vi "SR1-Test.vi"() -> ()   [LabVIEW 2014]
uses:
  Stanford Research SR1.lvlib
panel:
  in  "Start Button":bool
  out "Spectrum":cluster{dbl, dbl, dbl[]}(graph)
  in  "Read Button":bool
  in  "Stop Button":bool
  out "error out":errorcluster
  out "ID":string
  in  "VISA resource name":refnum<visa-resource-name>
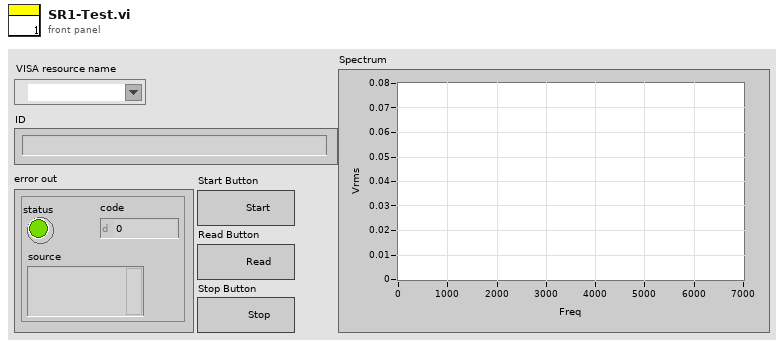
[diagram p1: front panel]
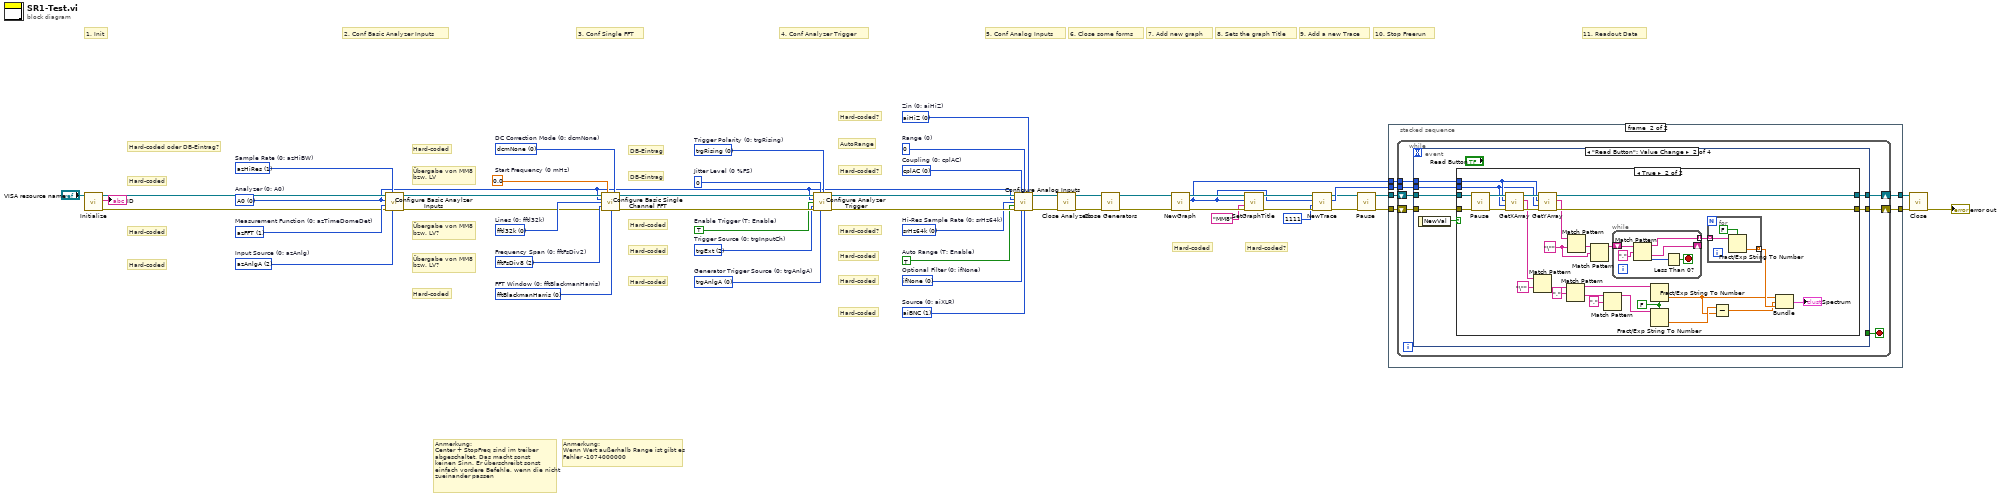
[diagram p0: block diagram]
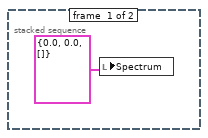
[diagram p2: hidden frame]
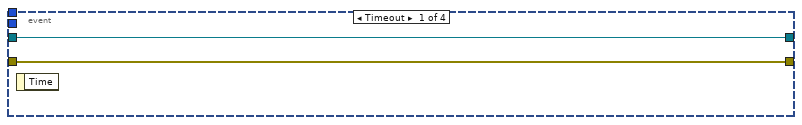
[diagram p3: hidden frame]
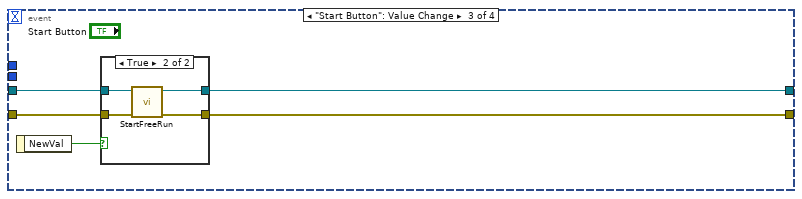
[diagram p5: hidden frame]
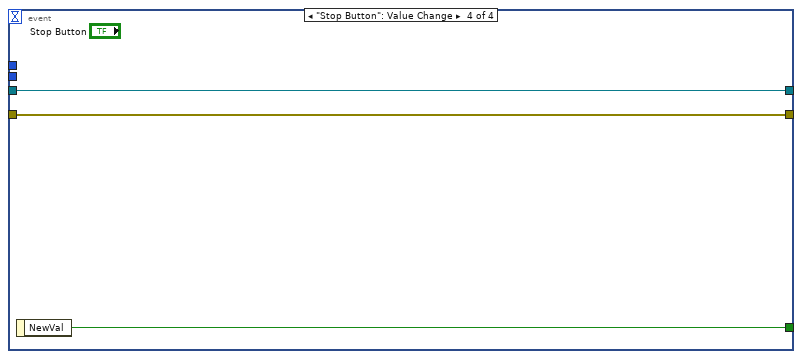
[diagram p7: hidden frame]
diagram:
  w22 = 0 items=["aiHiZ", "aiz300", "aiz600"]  # Zin (0: aiHiZ)
  w23 = 0  # Range (0)
  w24 = u16 0 items=["cplAC", "cplDC"]  # Coupling (0: cplAC)
  w25 = 1 items=["aiXLR", "aiBNC", "aiGenMon", "aiDigCommonMode"]  # Source (0: aiXLR)
  w26 = 0 items=["ifNone", "ifFiler1", "ifFilter2", "ifFilter3", "ifFilter4", "ifGround"]  # Optional Filter (0: ifNone)
  w27 = 0 items=["srHz64k", "srHz128k", "srOSR", "srOSRx2"]  # Hi-Res Sample Rate (0: srHz64k)
  w28 = TRUE  # Auto Range (T: Enable)
  w31 = 0 items=["trgAnlgA", "trgAnlgB", "trgDigA", "trgDigB", "trgJitter"]  # Generator Trigger Source (0: trgAnlgA)
  w32 = 2 items=["trgInputCh", "trgOtherCh", "trgExt", "trgManual", "trgGen", "trgDigAudBlock", "trgBurstA", "trgBurstB"]  # Trigger Source (0: trgInputCh)
  w33 = u16 0 items=["trgRising", "trgFalling"]  # Trigger Polarity (0: trgRising)
  w34 = 0  # Jitter Level (0 %FS)
  w35 = TRUE  # Enable Trigger (T: Enable)
  w40 = 1 items=["azHiBW", "azHiRes", "azISR", "azDetOutSR"]  # Sample Rate (0: azHiBW)
  w41 = 2 items=["azAnlg", "azDig", "azAnlgA", "azAnlgB", "azDigA", "azDigB", "azDetOut"]  # Input Source (0: azAnlg)
  w21 = 0 items=["A0", "A1"]  # Analyzer (0: A0)
  w42 = 1 items=["azTimeDomeDet", "azFFT", "azFFT2Ch", "azTHD", "azIMD", "azMultitone", "azJitter", "azHistogram", "azOctave"]  # Measurement Function (0: azTimeDomeDet)
  w45 = 0 items=["dcmNone", "dcmMean", "dcmPkPK"]  # DC Correction Mode (0: dcmNone)
  w46 = 0 items=["fftBlackmanHarris", "fftHann", "fftHamming", "fftEquiripple", "fftFlattop", "fftGaussian", "fftKaiser", "fftUniform", "fftRifeVincent4", "fftRifeVincent5", "fftRifeVincent10", "fftBlackmanHarris7", "fftVariable"]  # FFT Window (0: fftBlackmanHarris)
  w47 = 2 items=["fftFsDiv2", "fftFsDiv4", "fftFsDiv8", "fftFsDiv16", "fftFsDiv32", "fftFsDiv64", "fftFsDiv128", "fftFsDiv256", "fftFsDiv512", "fftFsDiv1024"]  # Frequency Span (0: fftFsDiv2)
  w48 = 0 items=["fftl32k", "fftl16k", "fftl8k", "fftl4k", "fftl2k", "fftl1k", "fftl512", "fftl256"]  # Lines (0: fftl32k)
  w49 = 0.0  # Start Frequency (0 mHz)
  # "11. Readout Data"
  # "10. Stop Freerun"
  # "Hard-coded"
  # "Hard-coded?"
  # "9. Add a new Trace"
  # "8. Sets the graph Title"
  # "7. Add new graph"
  # "6. Close some forms"
  # "5. Conf Analog Inputs"
  # "4. Conf Analyzer Trigger"
  # "3. Conf Single FFT"
  # "2. Conf Basic Analyzer Inputs"
  # "1. Init"
  # "Hard-coded"
  # "Hard-coded"
  # "Hard-coded"
  # "Hard-coded?"
  # "Hard-coded?"
  # "AutoRange"
  # "Hard-coded?"
  # "Hard-coded"
  # "Hard-coded"
  # "Hard-coded"
  # "DB-Eintrag"
  # "DB-Eintrag"
  # "Hard-coded"
  # "Übergabe von MM8\nbzw. LV?"
  # "Übergabe von MM8\nbzw. LV?"
  # "Übergabe von MM8\nbzw. LV"
  # "Hard-coded"
  # "Hard-coded"
  # "Hard-coded"
  # "Hard-coded"
  # "Hard-coded oder DB-Eintrag?"
  # "Anmerkung:\nWenn Wert außerhalb Range ist gibt es\nFehler -1074000000"
  # "Anmerkung:\nCenter + StopFreq sind im treiber\nabgeschaltet. Das macht sonst \nkeinen Sinn. Er überschreibt sonst\neinfach vordere Befehle, wenn die nicht\nzueinander passen"
  n1 = call "Initialize.vi"("VISA resource name"="VISA resource name") -> ("error out"=w38:errorcluster, "ID"=→"ID":string, "VISA resource name out"=w39:refnum<visa-resource-name>)  [unwired: 8 in]
  n2 = call "Configure Basic Anaylzer Inputs.vi"("Input Source (0: azAnlg)"=w41, "Sample Rate (0: azHiBW)"=w40, "error in (no error)"=w38, "Measurement Function (0: azTimeDomeDet)"=w42, "Analyzer (0: A0)"=w21, "VISA resource name"=w39) -> ("error out"=w44:errorcluster, "VISA resource name out"=w43:refnum<visa-resource-name>)  [unwired: 4 in]
  n3 = call "Configure Basic Single Channel FFT .vi"("VISA resource name"=w43, "Start Frequency (0 mHz)"=w49, "DC Correction Mode (0: dcmNone)"=w45, "Analyzer (0: A0)"=w21, "Lines (0: fftl32k)"=w48, "Frequency Span (0: fftFsDiv2)"=w47, "error in (no error)"=w44, "FFT Window (0: fftBlackmanHarris)"=w46) -> ("VISA resource name out"=w36:refnum<visa-resource-name>, "error out"=w37:errorcluster)  [unwired: 6 in]
  n4 = call "Configure Analyzer Trigger.vi"("VISA resource name"=w36, "Jitter Level (0 %FS)"=w34, "Trigger Polarity (0: trgRising)"=w33, "Analyzer (0: A0)"=w21, "Enable Trigger (T: Enable)"=w35, "Trigger Source (0: trgInputCh)"=w32, "error in (no error)"=w37, "Generator Trigger Source (0: trgAnlgA)"=w31) -> ("VISA resource name out"=w29:refnum<visa-resource-name>, "error out"=w30:errorcluster)  [unwired: 6 in]
  n5 = call "Configure Analog Inputs.vi"("VISA resource name"=w29, "Coupling (0: cplAC)"=w24, "Range (0)"=w23, "Zin (0: aiHiZ)"=w22, "Channel (0: ChannelA)"=w21, "Hi-Res Sample Rate (0: srHz64k)"=w27, "Auto Range (T: Enable)"=w28, "error in (no error)"=w30, "Optional Filter (0: ifNone)"=w26, "Source (0: aiXLR)"=w25) -> ("VISA resource name out"=w18:refnum<visa-resource-name>, "error out"=w17:errorcluster)  [unwired: 4 in]
  n6 = call "Close Analyzers.vi"("error in (no error)"=w17, "VISA resource name"=w18) -> ("error out"=w20:errorcluster, "VISA resource name out"=w19:refnum<visa-resource-name>)  [unwired: 8 in]
  n7 = call "Close Generators.vi"("error in (no error)"=w20, "VISA resource name"=w19) -> ("error out"=w16:errorcluster, "VISA resource name out"=w15:refnum<visa-resource-name>)  [unwired: 8 in]
  n8 = call "NewGraph.vi"("error in (no error)"=w16, "VISA resource name"=w15) -> ("error out"=w12:errorcluster, "GraphID"=w6:i32, "VISA resource name out"=w11:refnum<visa-resource-name>)  [unwired: 7 in]
  n9 = call "SetGraphTitle.vi"("error in (no error)"=w12, "Title"="MM8", "GraphID"=w6, "VISA resource name"=w11) -> ("error out"=w13:errorcluster, "VISA resource name out"=w14:refnum<visa-resource-name>)  [unwired: 6 in]
  n10 = call "NewTrace.vi"("error in (no error)"=w13, "TraceType"=1111, "GraphID"=w6, "VISA resource name"=w14) -> ("error out"=w4:errorcluster, "TraceID"=w5:i32, "VISA resource name out"=w2:refnum<visa-resource-name>)  [unwired: 5 in]
  n11 = call "Pause.vi"("error in (no error)"=w4, "VISA resource name"=w2) -> ("error out"=w3:errorcluster, "VISA resource name out"=w1:refnum<visa-resource-name>)  [unwired: 8 in]
  n12 = stacked-sequence {
    tunnel: [_ w59] -> w8
    tunnel: [_ w58] -> w7
    tunnel: w6 -> [_ w57]
    tunnel: w5 -> [_ w56]
    tunnel: w3 -> [_ w55]
    tunnel: w1 -> [_ w54]
    frame #0 {
      n13 = local write "Spectrum"(cluster{dbl, dbl, dbl[]} {0.0, 0.0, []} ("Spectrum")) -> ()
    }
    frame #1 {
      n14 = while {
        shift-right: [w63] -> w58
        shift-left: w54 -> [w62]
        shift-right: [w64] -> w59
        shift-left: w55 -> [w65]
        tunnel: w57 -> [w61]
        tunnel: w56 -> [w60]
        stop <- w66 stop-if-true
        n15 = event shown="[1] \"Read Button\": Value Change" {
          selector: _ -> [_ _ _ _]
          dyn-events: _ -> [_ _ _ _]
          timeout: _ -> [_ _ _ _]
          tunnel: [_ _ _ w129] -> w66
          tunnel: w65 -> [w68 w74 w119 w128]
          tunnel: [w68 w72 w116 w128] -> w64
          tunnel: [w67 w71 w117 w127] -> w63
          tunnel: w62 -> [w67 w73 w120 w127]
          tunnel: w61 -> [_ w70 _ _]
          tunnel: w60 -> [_ w69 _ _]
          event Timeout {
            n16 = event-data() -> ()  [unwired: 1 in, 1 out]
          }
          event "Read Button": Value Change {
            n17 = event-data() -> ("NewVal"=w75:bool)  [unwired: 1 in]
            n18 = case shown="True" w75 {
              tunnel: w74 -> [w76 w106]
              tunnel: w73 -> [w77 w105]
              tunnel: [w76 w101] -> w72
              tunnel: [w77 w99] -> w71
              tunnel: w70 -> [_ w98]
              tunnel: w69 -> [_ w97]
              frame False {
              }
              frame True {
                w83 = FALSE ("use system decimal point (T)")
                w96 = "\"" ("regular expression")
                n19 = call "Pause.vi"("error in (no error)"=w106, "VISA resource name"=w105) -> ("error out"=w103:errorcluster, "VISA resource name out"=w104:refnum<visa-resource-name>)  [unwired: 8 in]
                n20 = call "GetXArray.vi"("error in (no error)"=w103, "TraceID"=w97, "GraphID"=w98, "VISA resource name"=w104) -> ("error out"=w102:errorcluster, "xArray"=w90:string, "VISA resource name out"=w100:refnum<visa-resource-name>)  [unwired: 5 in]
                n21 = Match Pattern(string=w90, regular expression="\"") -> (after substring=w89:string)  [unwired: 1 in, 3 out]
                n22 = call "GetYArray.vi"("error in (no error)"=w102, "TraceID"=w97, "GraphID"=w98, "VISA resource name"=w100) -> ("error out"=w101:errorcluster, "yArray"=w93:string, "VISA resource name out"=w99:refnum<visa-resource-name>)  [unwired: 5 in]
                n23 = Match Pattern(string=w89, regular expression=",") -> (before substring=w85:string, after substring=w86:string)  [unwired: 1 in, 2 out]
                n24 = Match Pattern(string=w93, regular expression=w96) -> (after substring=w94:string)  [unwired: 1 in, 3 out]
                n25 = Match Pattern(string=w94, regular expression=w96) -> (before substring=w95:string)  [unwired: 1 in, 3 out]
                n26 = Match Pattern(string=w86, regular expression=",") -> (before substring=w84:string)  [unwired: 1 in, 3 out]
                n27 = while {
                  tunnel: [w110] -> w92 mode=indexing
                  shift-right: [w109] -> _
                  shift-left: w95 -> [w112]
                  stop <- w107 stop-if-true
                  n28 = Match Pattern(string=w112, regular expression=",") -> (before substring=w110:string, after substring=w109:string, offset past match=w108:i32)  [unwired: 1 in, 1 out]
                  n29 = Less Than 0?(x=w108) -> (x < 0?=w107:bool)
                }
                n30 = Fract/Exp String To Number(use system decimal point (T)=w83, string=w85) -> (number=w79:dbl)  [unwired: 2 in, 1 out]
                n31 = Fract/Exp String To Number(use system decimal point (T)=w83, string=w84) -> (number=w80:dbl)  [unwired: 2 in, 1 out]
                n32 = for {
                  tunnel: w92 -> [w115] mode=indexing
                  tunnel: [w113] -> w82 mode=indexing
                  n33 = Fract/Exp String To Number(use system decimal point (T)=FALSE, string=w115) -> (number=w113:dbl)  [unwired: 2 in, 1 out]
                }
                n34 = Subtract(x=w80, y=w79) -> (x-y=w78:dbl)
                n35 = Bundle(w79, w78, w82) -> (→"Spectrum":cluster{dbl, dbl, dbl[]})  [unwired: 1 in]
              }
            }
          }
          event "Start Button": Value Change {
            n36 = event-data() -> ("NewVal"=w118:bool)  [unwired: 1 in]
            n37 = case shown="True" w118 {
              tunnel: w120 -> [w122 w126]
              tunnel: w119 -> [w121 w125]
              tunnel: [w122 w124] -> w117
              tunnel: [w121 w123] -> w116
              frame False {
              }
              frame True {
                n38 = call "StartFreeRun.vi"("error in (no error)"=w125, "VISA resource name"=w126) -> ("error out"=w123:errorcluster, "VISA resource name out"=w124:refnum<visa-resource-name>)  [unwired: 8 in]
              }
            }
          }
          event "Stop Button": Value Change {
            n39 = event-data() -> ("NewVal"=w129:bool)  [unwired: 1 in]
          }
        }
      }
    }
  }
  n40 = call "Close.vi"("error in (no error)"=w8, "VISA resource name"=w7) -> ("error out"=→"error out":errorcluster)  [unwired: 9 in]
